vi "Invalid Reference Error.vi"() -> (0 "error out":errorcluster)   [LabVIEW 2017, in "Composed Log.lvlib" / "LoggerReference.lvclass"]
uses:
  LoggerReference.lvclass
  <vilib>/Utility/error.llb/Error Cluster From Error Code.vi
  <vilib>/ErrorRing/Error Ring.xnode
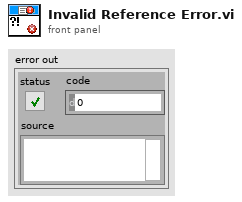
[diagram p1: front panel]
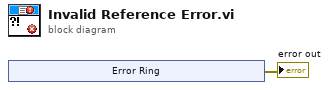
[diagram p0: block diagram]
diagram:
  n1 = xnode "Error Ring"() -> ("error out"=→"error out":errorcluster)
